vi "Main.vi"   [LabVIEW 2020]
panel:
  # "Get Psyched!"
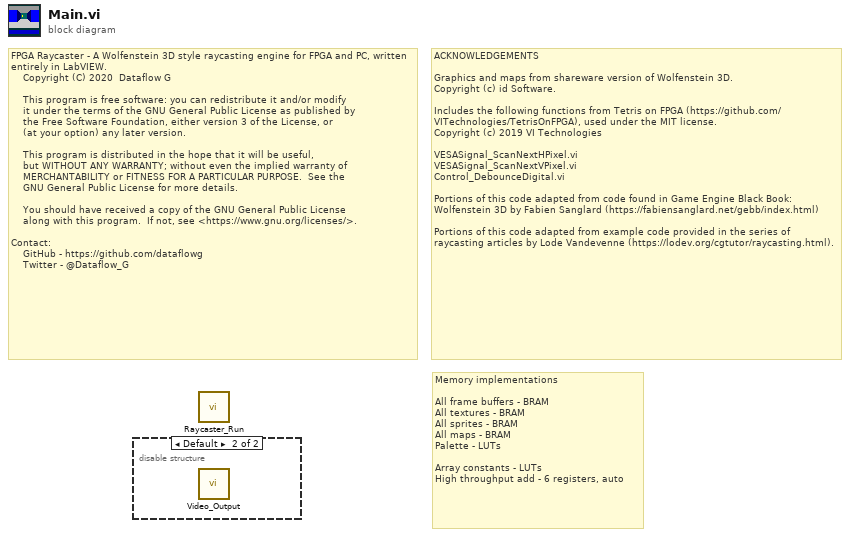
[diagram p0: block diagram]
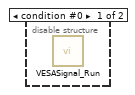
[diagram p2: hidden frame]
diagram:
  # "ACKNOWLEDGEMENTS\n\nGraphics and maps from shareware version of Wolfenstein 3D.\nCopyright (c) id Software.\n\nIncludes the following functions from Tetris on FPGA (https://github.com/VITechnologies/TetrisOnFPGA), used under the MIT license.\nCopyright (c) 2019 VI Technologies\n\nVESASignal_ScanNextHPixel.vi\nVESASignal_ScanNextVPixel.vi\nControl_DebounceDigital.vi\n\nPortions of this code adapted from code found in Game Engine Black Book: Wolfenstein 3D by Fabien Sanglard (https://fabiensanglard.net/gebb/index.html)\n\nPortions of this code adapted from example code provided in the series of raycasting articles by Lode Vandevenne (https://lodev.org/cgtutor/raycasting.html)."
  # "FPGA Raycaster - A Wolfenstein 3D style raycasting engine for FPGA and PC, written entirely in LabVIEW.\n    Copyright (C) 2020  Dataflow G\n    \n    This program is free software: you can redistribute it and/or modify\n    it under the terms of the GNU General Public License as published by\n    the Free Software Foundation, either version 3 of the License, or\n    (at your option) any later version.\n\n    This program is distributed in the hope that it will be useful,\n    but WITHOUT ANY WARRANTY; without even the implied warranty of\n    MERCHANTABILITY or FITNESS FOR A PARTICULAR PURPOSE.  See the\n    GNU General Public License for more details.\n\n    You should have received a copy of the GNU General Public License\n    along with this program.  If not, see <https://www.gnu.org/licenses/>.\n\nContact:\n    GitHub - https://github.com/dataflowg\n    Twitter - @Dataflow_G"
  # "Memory implementations\n\nAll frame buffers - BRAM\nAll textures - BRAM\nAll sprites - BRAM\nAll maps - BRAM\nPalette - LUTs\n\nArray constants - LUTs\nHigh throughput add - 6 registers, auto"
  n1 = disable-structure shown="Default" {
    frame condition #0 {
      n2 = call "VESASignal_Run.vi"() -> ()  [unwired: 12 in]
    }
    frame condition #1 (active) {
      n3 = call "Video_Output.vi"() -> ()  [unwired: 12 in]
    }
  }
  n4 = call "Raycaster_Run.vi"() -> ()  [unwired: 12 in]
